vi "PrintDiploma.vi"(8 "error in (no error)":errorcluster, 9 "printer name (default)":string="CutePDF Writer", 10 "Path":path, 11 "Diploma":T1={"Name"="", "Swim Length"="", "With Aids"=TRUE, "Date"=timestamp(0 s since 1904-01-01), "Unit"=""}) -> (0 "error out":errorcluster)   [LabVIEW 2018]
uses:
  TypeDef/Diploma.ctl
  <vilib>/addons/_office/word.llb/Word Find & Replace (str).vi
  <vilib>/Utility/NIReport.llb/NI_report.lvclass
  <vilib>/addons/_office/NI_ReportGenerationToolkit.lvlib
  <vilib>/Utility/NIReport.llb/Word/NI_Word.lvclass
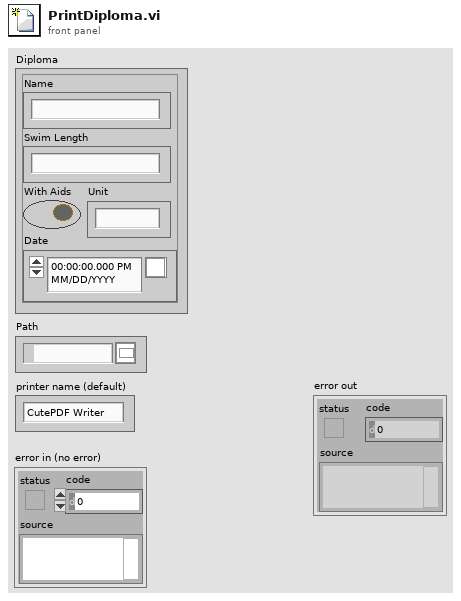
[diagram p1: front panel]
types:
  T1 = typedef "Diploma.ctl" = cluster{"Name":string, "Swim Length":string, "With Aids":bool, "Date":timestamp, "Unit":string}
  T2 = enum16{"Standard Report", "HTML", "Word", "Excel"}
  T3 = enum16{"maximized", "minimized", "normal", "no change"}
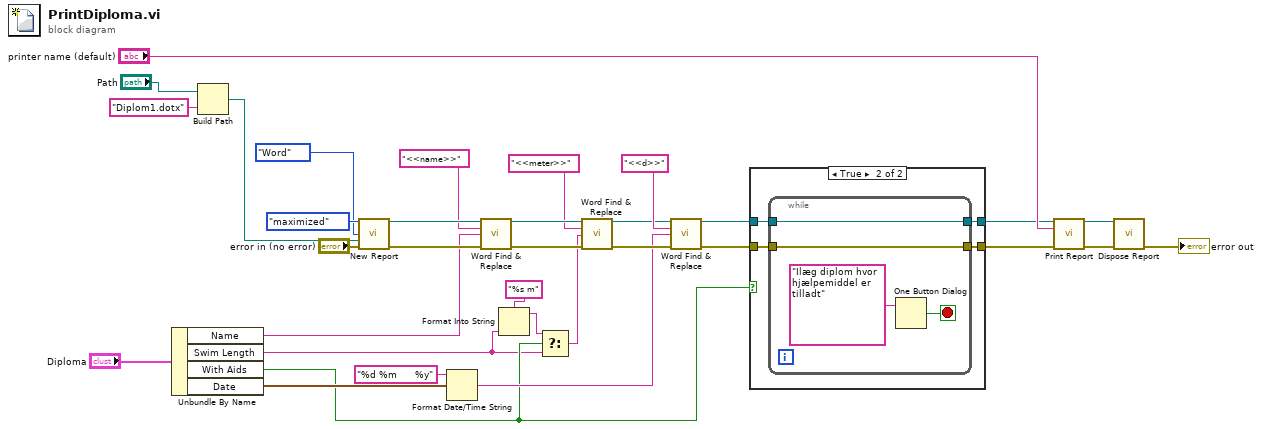
[diagram p0: block diagram]
diagram:
  n1 = Unbundle By Name("Diploma") -> ("Name"=w23:string, "Swim Length"=w3:string, "With Aids"=w5:bool, "Date"=w11:timestamp)
  n2 = Build Path(base path="Path", name or relative path="Diplom1.dotx") -> (appended path=w13:path)
  n3 = call <vilib>:"New Report.vi"("window state (normal)"=T3."maximized", "report type"=T2."Word", "template (empty)"=w13, "error in (no error)"="error in (no error)") -> ("report out"=w32:refnum<class "NI_report.lvclass">, "error out"=w31:errorcluster)  [unwired: 10 in]
  n4 = Format Date/Time String(time format string (%c)="%d %m      %y", seconds (now)=w11) -> (date/time string=w9:string)  [unwired: 1 in]
  n5 = call-poly <vilib>:"Word Find & Replace.vi"("report in"=w32, "find what?"="<<name>>", "replace with"=w23, "error in (no error)"=w31) -> ("report out"=w29:refnum<class "NI_report.lvclass">, "error out"=w28:errorcluster)  [unwired: 9 in, 1 out]
  n6 = Format Into String(format string="%s m", w3) -> (resulting string=w1:string)  [unwired: 2 in, 1 out]
  n7 = Select(t=w1, s=w5, f=w3) -> (s? t:f=w4:string)
  n8 = call-poly <vilib>:"Word Find & Replace.vi"("report in"=w29, "find what?"="<<meter>>", "replace with"=w4, "error in (no error)"=w28) -> ("report out"=w21:refnum<class "NI_report.lvclass">, "error out"=w20:errorcluster)  [unwired: 9 in, 1 out]
  n9 = call-poly <vilib>:"Word Find & Replace.vi"("report in"=w21, "find what?"="<<d>>", "replace with"=w9, "error in (no error)"=w20) -> ("report out"=w18:refnum<class "NI_report.lvclass">, "error out"=w19:errorcluster)  [unwired: 9 in, 1 out]
  n10 = case shown="True" w5 {
    tunnel: w19 -> [w34 w39]
    tunnel: w18 -> [w35 w38]
    tunnel: [w35 w37] -> w17
    tunnel: [w34 w36] -> w16
    frame False {
    }
    frame True {
      n11 = while {
        tunnel: w39 -> [w42]
        tunnel: w38 -> [w43]
        tunnel: [w43] -> w37
        tunnel: [w42] -> w36
        stop <- w41 stop-if-true
        n12 = One Button Dialog(message="Ilæg diplom hvor hjælpemiddel er tilladt") -> (true=w41:bool)  [unwired: 1 in]
      }
    }
  }
  n13 = call-dynamic "Print Report.vi"("report in"=w17, "printer name (default)"="printer name (default)", "error in (no error)"=w16) -> ("report out"=w7:refnum<class "NI_report.lvclass">, "error out"=w8:errorcluster)  [unwired: 11 in]
  n14 = call-dynamic "Dispose Report.vi"("report in"=w7, "error in (no error)"=w8) -> ("error out"=→"error out":errorcluster)  [unwired: 13 in]
